vi "Beam Chopper.vi"(2 "Samples per toggle":dbl=6.0, 10 "Milliseconds per sample":u32=500, 11 "stop":bool) -> (0 "Current Sample":dbl, 8 "Boolean":bool)   [LabVIEW 2017]
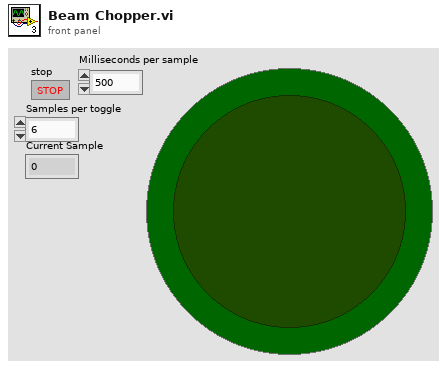
[diagram p1: front panel]
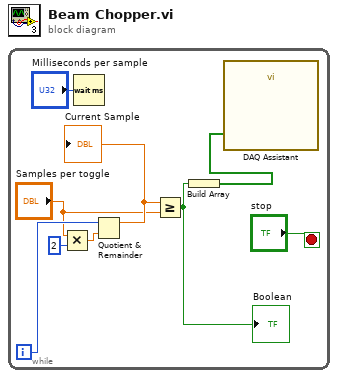
[diagram p0: block diagram]
diagram:
  n1 = while {
    i -> [w5]
    stop <- "stop" stop-if-true
    n2 = Multiply(x="Samples per toggle", y=2) -> (x*y=w8:dbl)
    n3 = Wait (ms)(milliseconds to wait="Milliseconds per sample") -> ()  [unwired: 1 out]
    n4 = Quotient & Remainder(x=w5, y=w8) -> (x-y*floor(x/y)=w6:dbl)  [unwired: 1 out]
    "Current Sample" <- w6
    n5 = Greater Or Equal?(x=w6, y="Samples per toggle") -> (x >= y?=w1:bool)
    "Boolean" <- w1
    n6 = Build Array(w1) -> (w2:bool[])
    n7 = call "DAQ Assistant"("data"=w2) -> ()  [unwired: 17 in, 2 out]
  }
